vi "DenoiseFIlter.vi"(3 "error in (no error)":errorcluster, 4 "Filter Level":i32, 5 "Signal Input":bool) -> (0 "error out":errorcluster, 1 "Post-Filter":i16(graph), 2 "Signal Output":bool)   [LabVIEW 2020]
panel:
  out "Pre-Filter":i16(graph)
  # "Leave these as is, they are for the wire input and output for\nthe sub-vi"
  # "Change this to be the number of points that you want to check\nfor the filter"
  # "Two charts for a sid-by-side comparison to make sure that the signal is being filtered enough"
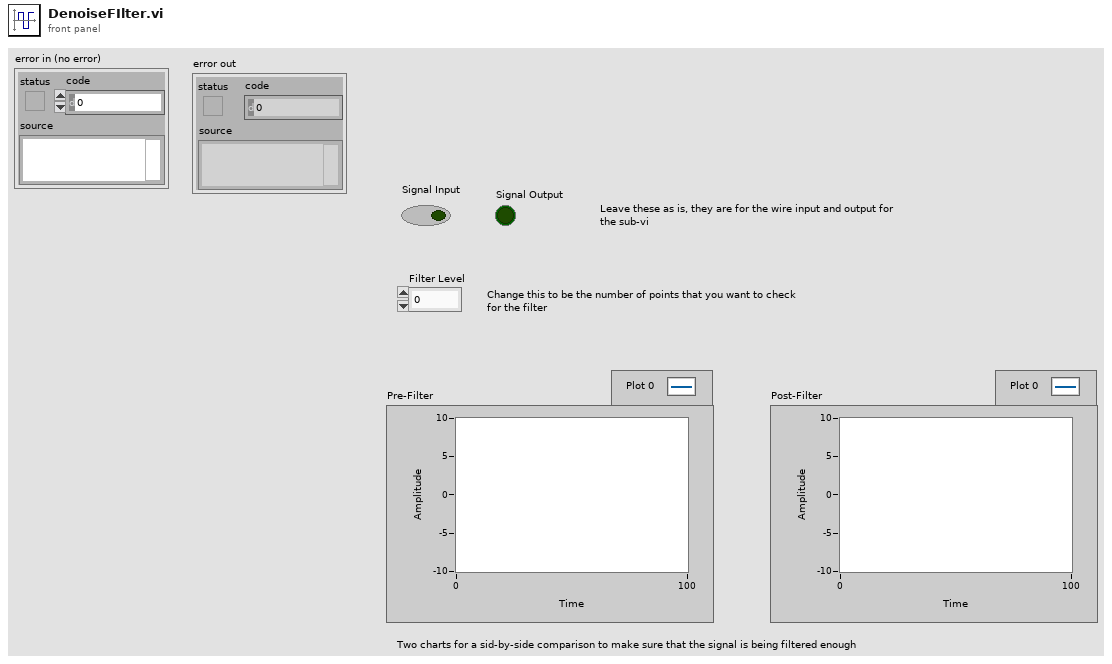
[diagram p1: front panel]
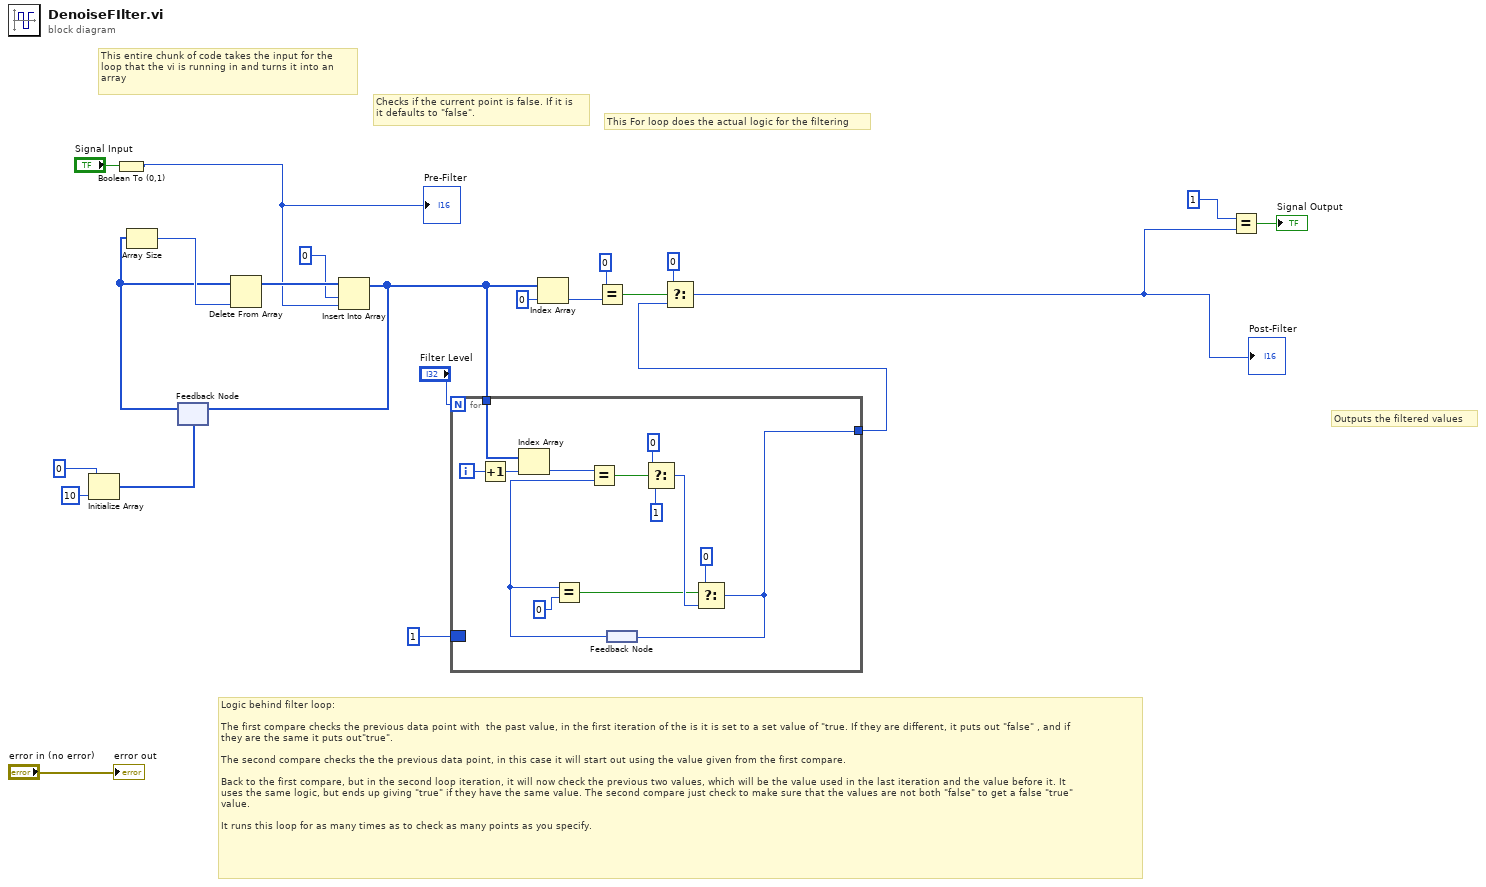
[diagram p0: block diagram]
diagram:
  # "Logic behind filter loop:\n\nThe first compare checks the previous data point with  the past value, in the first iteration of the is it is set to a set value of \"true. If they are different, it puts out \"false\" , and if \nthey are the same it puts out\"true\".\n\nThe second compare checks the the previous data point, in this case it will start out using the value given from the first compare.\n\nBack to the first compare, but in the second loop iteration, it will now check the previous two values, which will be the value used in the last iteration and the value before it. It \nuses the same logic, but ends up giving \"true\" if they have the same value. The second compare just check to make sure that the values are not both \"false\" to get a false \"true\"\nvalue.\n\nIt runs this loop for as many times as to check as many points as you specify."
  # "Checks if the current point is false. If it is\nit defaults to \"false\"."
  # "Outputs the filtered values"
  # "This entire chunk of code takes the input for the\nloop that the vi is running in and turns it into an \narray"
  # "This For loop does the actual logic for the filtering"
  n1 = Initialize Array(i16 0 ("element"), 10 ("dimension size")) -> (w22:i16[])
  n2 = Boolean To (0,1)(Boolean="Signal Input") -> (0, 1=w4:i16)
  "Pre-Filter" <- w4
  n3 = feedback #1(w22) -> (w18:i16[])
  n4 = Array Size(array=w18) -> (size(s)=w19:i32)
  n5 = Delete From Array(array=w18, index=w19) -> (array with subset deleted=w17:i16[])  [unwired: 1 in, 1 out]
  n6 = Insert Into Array(array=w17, index=0, new element=w4) -> (w9:i16[])
  n7 = feedback-in #1(w9) -> ()
  n8 = for {
    N: "Filter Level" -> [_]
    tunnel: w9 -> [w35]
    border: i16 1 -> [_]
    tunnel: [w27] -> w7
    i -> [w34]
    n9 = Increment(x=w34) -> (x+1=w33:i32)
    n10 = Index Array(array=w35, index=w33) -> (element=w32:i16)
    n11 = feedback #2() -> (w25:i16)
    n12 = Equal?(x=w25, y=i16 0) -> (x = y?=w23:bool)
    n13 = Equal?(x=w32, y=w25) -> (x = y?=w31:bool)
    n14 = Select(t=i16 0, s=w31, f=i16 1) -> (s? t:f=w26:i16)
    n15 = Select(t=i16 0, s=w23, f=w26) -> (s? t:f=w27:i16)
    n16 = feedback-in #2(w27) -> ()
  }
  n17 = Index Array(array=w9, index=0) -> (element=w14:i16)
  n18 = Equal?(x=i16 0, y=w14) -> (x = y?=w12:bool)
  n19 = Select(t=i16 0, s=w12, f=w7) -> (s? t:f=w3:i16)
  "Post-Filter" <- w3
  n20 = Equal?(x=i16 1, y=w3) -> (x = y?=→"Signal Output":bool)
  "error out" <- "error in (no error)"
